vi "GetDoubleFeatureValue.vi"(9 "pFeatureName":string, 10 "handle":i64, 11 "error in (no error)":errorcluster) -> (2 "pDoubleValue":dbl, 3 "error out":errorcluster)   [LabVIEW 2016]
uses:
  MVSDKmd.dll
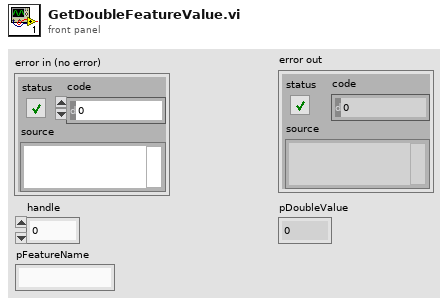
[diagram p1: front panel]
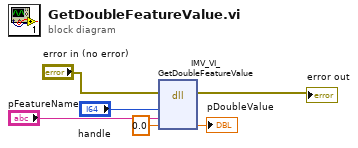
[diagram p0: block diagram]
diagram:
  n1 = dll-call lib="MVSDKmd.dll" fn="IMV_VI_GetDoubleFeatureValue"(error in="error in (no error)", "handle"="handle", "pFeatureName"="pFeatureName", "pDoubleValue"=0.0) -> (error out=→"error out":errorcluster, "pDoubleValue"=→"pDoubleValue":dbl)  [unwired: 5 in, 1 out]
